vi "captTemperature.vi"(8 "error in":errorcluster) -> (0 "error out 2":errorcluster caption="error out", 2 "Value":dbl)   [LabVIEW 2012]
uses:
  GlobalVariables/GantnerParameters.vi
  GlobalVariables/CommunicationActivity.vi
  ISMBUS32.DLL
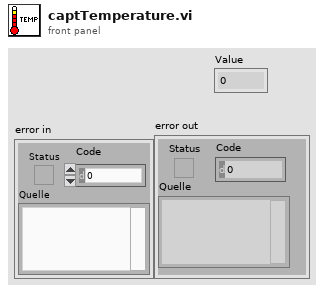
[diagram p1: front panel]
types:
  T1 = typedef "ISMBUS_Module.ctl" = cluster{"ModuleAddress":i32, "ModuleKindIndex":i32, "ModuleKind":string, " Protocol":string, " BaudRate":i32, "CharFormat":string, "BaudRateIndex":i32, "FormatIndex":i32, "ProtocolIndex":i32, "Location":string, "SerialNumber":string, "Vendor":string, "HWRelease":string, "SWRelease":string, "ControllerType":string, "ChannelList":T2[], "ChannelCount":i32, " COM Port":i32}
  T2 = typedef "ISMBUS_Channel.ctl" = cluster{" Description":string, " ChannelKindIndex":i32, "ChannelFormatIndex":i32, " FieldLength":i32, "Precision":i32, "Unit":string, "Mode":i32}
  T3 = cluster{"Module":T1, "PT01 chanel":u32, "Temperature chanel":u32, "HEV01 chanel":u32, "HEV02 chanel":u32, "PressureLimit":dbl}
  T4 = cluster{"KellerActive":bool, "GantnerActive":bool, "BrooksActive":bool}
  T5 = cluster{"KellerActive":bool, bool, "BrooksActive":bool}
  T6 = cluster{bool, "GantnerActive":bool, "BrooksActive":bool}
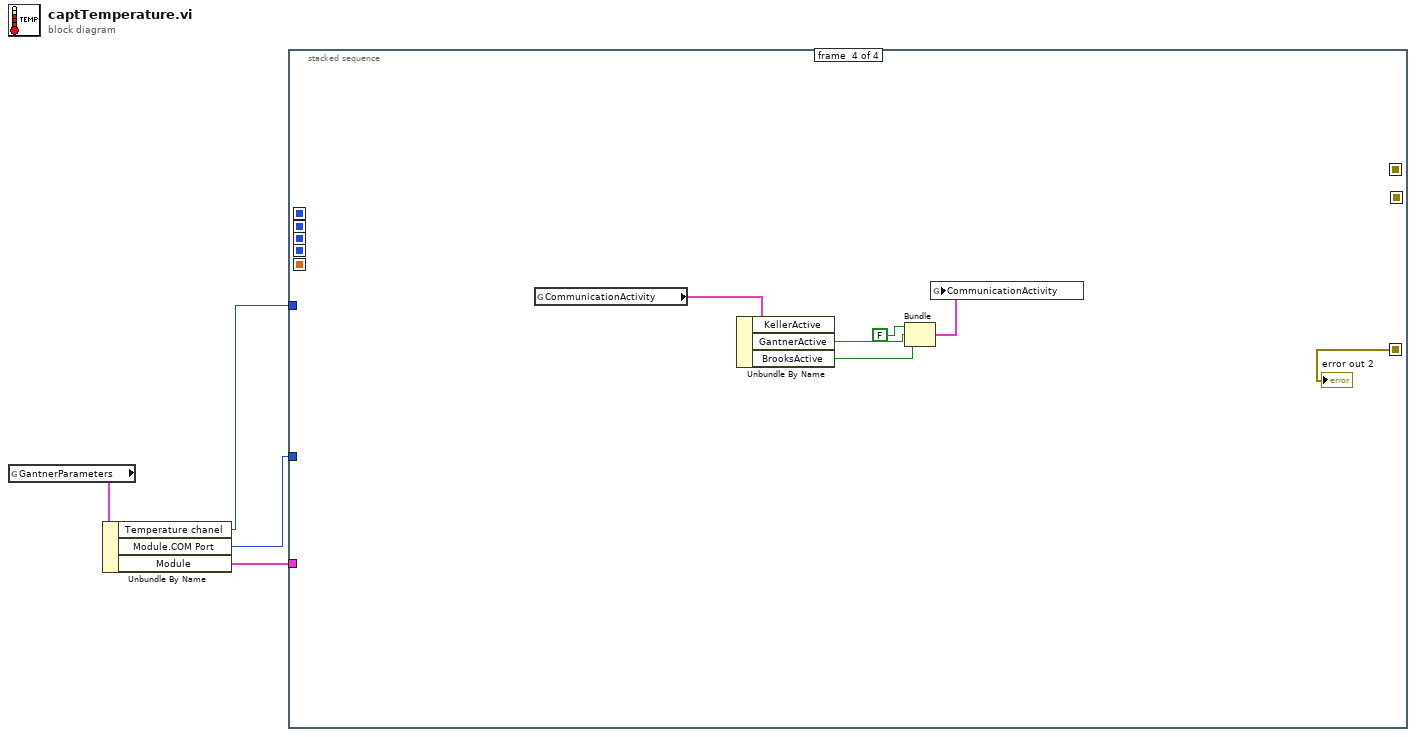
[diagram p0: block diagram]
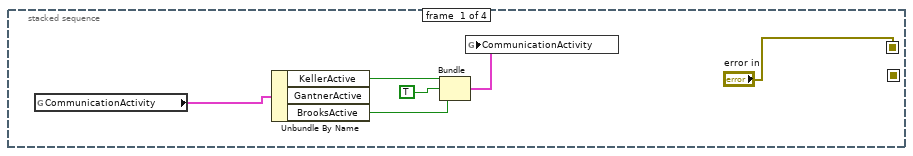
[diagram p2: hidden frame]
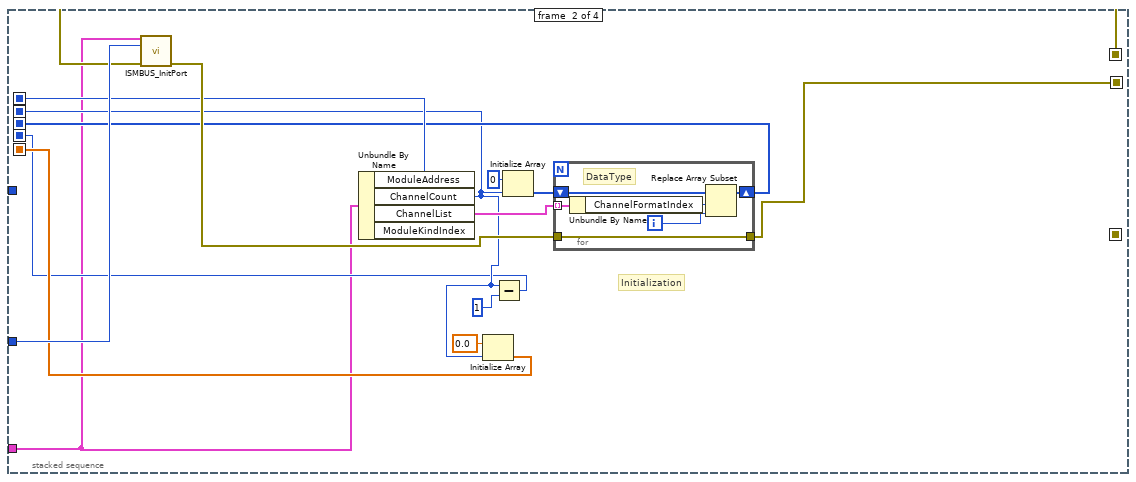
[diagram p3: hidden frame]
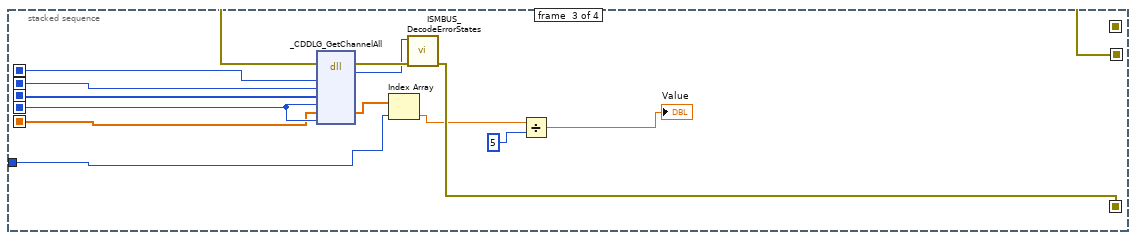
[diagram p4: hidden frame]
diagram:
  n1 = global read "GantnerParameters.vi" "GantnerParameters"() -> (w4:T3)
  n2 = Unbundle By Name(w4) -> ("Temperature chanel"=w1:u32, "Module.COM Port"=w3:i32, "Module"=w2:T1)
  n3 = stacked-sequence {
    seq-local: ["error in" _ _ _] -> [_ w24 _ _]
    seq-local: [_ _ w35 _] -> [_ _ _ w51]
    seq-local: [_ w17 _ _] -> [_ _ w42 _]
    seq-local: [_ w16 _ _] -> [_ _ w41 _]
    seq-local: [_ w13 _ _] -> [_ _ w40 _]
    seq-local: [_ w15 _ _] -> [_ _ w39 _]
    seq-local: [_ w12 _ _] -> [_ _ w38 _]
    seq-local: [_ w14 _ _] -> [_ _ w37 _]
    tunnel: w3 -> [_ w25 _ _]
    tunnel: w2 -> [_ w11 _ _]
    tunnel: w1 -> [_ _ w36 _]
    frame #0 {
      n4 = global read "CommunicationActivity.vi" "CommunicationActivity"() -> (w10:T4)
      n5 = Unbundle By Name(w10) -> ("KellerActive"=w6:bool, "BrooksActive"=w8:bool)  [unwired: 1 out]
      n6 = Bundle("KellerActive"=w6, TRUE, "BrooksActive"=w8) -> (w9:T5)  [unwired: 1 in]
      n7 = global write "CommunicationActivity.vi" "CommunicationActivity"(w9) -> ()
    }
    frame #1 {
      # "Initialization"
      n8 = call "ISMBUS_InitPort.vi"("Module"=w11, "ComPort"=w25, "Fehler (Eingang - kein Fehler)"=w24) -> ("Fehler (Ausgang)"=w18:errorcluster)  [unwired: 12 out]
      n9 = Unbundle By Name(w11) -> ("ModuleAddress"=w16:i32, "ChannelCount"=w13:i32, "ChannelList"=w21:T2[])  [unwired: 1 out]
      n10 = Initialize Array(0.0, w13) -> (w14:dbl[])
      n11 = Subtract(x=w13, y=1) -> (x-y=w12:i32)
      n12 = Initialize Array(0 ("Element"), w13) -> (w22:i32[])
      n13 = for {
        tunnel: w21 -> [w30] mode=indexing
        shift-right: [w28] -> w15
        shift-left: w22 -> [w27]
        tunnel: w18 -> [w26]
        tunnel: [w26] -> w17
        i -> [w31]
        # "DataType"
        n14 = Unbundle By Name(w30) -> ("ChannelFormatIndex"=w29:i32)
        n15 = Replace Array Subset(array=w27, new element=w29, index=w31) -> (w28:i32[])
      }
    }
    frame #2 {
      n16 = dll-call lib="ISMBUS32.DLL" fn="_CDDLG_GetChannelAll"(error in=w42, "Address"=w41, "NumCh"=w40, "ArrDataTypes"=w39, "ArrDataTypeItemsSub1"=w38, "ArrValues"=w37, "ArrValuesItemsSub1"=w38) -> (error out=w45:errorcluster, w44:i32, "ArrValues"=w43:dbl[])  [unwired: 7 in, 1 out]
      n17 = Index Array(array=w43, index=w36) -> (element=w34:dbl)
      n18 = call "ISMBUS_DecodeErrorStates.vi"("Fehler (Eingang - kein Fehler)"=w45, "ISMBUS_Error State"=w44) -> ("Fehler (Ausgang)"=w35:errorcluster)  [unwired: 1 in, 8 out]
      n19 = Divide(x=w34, y=5) -> (x/y=→"Value":dbl)
    }
    frame #3 {
      n20 = global read "CommunicationActivity.vi" "CommunicationActivity"() -> (w50:T4)
      n21 = Unbundle By Name(w50) -> ("GantnerActive"=w46:bool, "BrooksActive"=w47:bool)  [unwired: 1 out]
      n22 = Bundle(FALSE, "GantnerActive"=w46, "BrooksActive"=w47) -> (w49:T6)  [unwired: 1 in]
      n23 = global write "CommunicationActivity.vi" "CommunicationActivity"(w49) -> ()
      "error out 2" <- w51
    }
  }
